vi "HEWH Round UEF.vi"(11 "Unrounded Value":dbl) -> (3 "Rounded Value":dbl format="%_3g")   [LabVIEW 2023]
panel:
  out "output variable":dbl
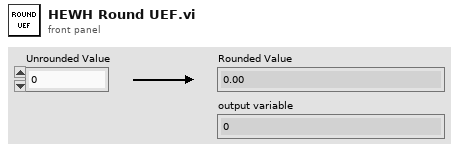
[diagram p1: front panel]
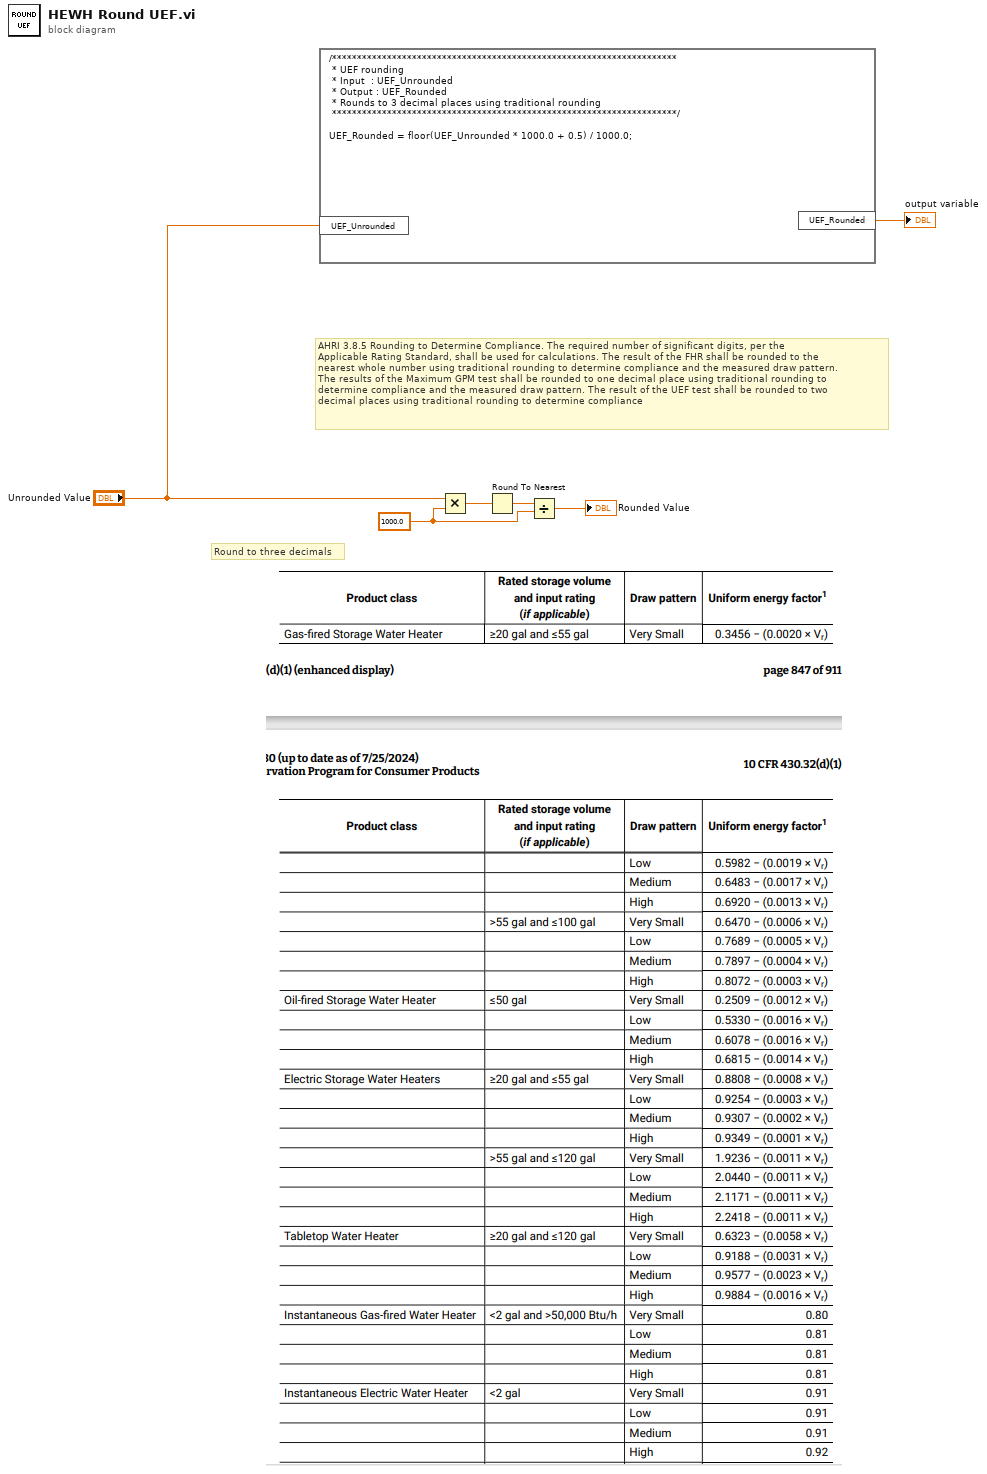
[diagram p0: block diagram]
diagram:
  w3 = 1000.0 ("y")
  # "Round to three decimals"
  # "AHRI 3.8.5 Rounding to Determine Compliance. The required number of significant digits, per the \nApplicable Rating Standard, shall be used for calculations. The result of the FHR shall be rounded to the \nnearest whole number using traditional rounding to determine compliance and the measured draw pattern. \nThe results of the Maximum GPM test shall be rounded to one decimal place using traditional rounding to \ndetermine compliance and the measured draw pattern. The result of the UEF test shall be rounded to two \ndecimal places using traditional rounding to determine compliance"
  n1 = formula code="/*********************************************************************\n * UEF rounding\n * Input  : UEF_Unrounded\n * Output : UEF_Rounded\n * Rounds to 3 decimal places using traditional rounding\n *********************************************************************/\n\nUEF_Rounded = floor(UEF_Unrounded * 1000.0 + 0.5) / 1000.0;"("UEF_Unrounded"="Unrounded Value") -> ("UEF_Rounded"=→"output variable":dbl)
  n2 = Multiply(x="Unrounded Value", y=w3) -> (x*y=w5:dbl)
  n3 = Round To Nearest(number=w5) -> (nearest integer value=w4:dbl)
  n4 = Divide(x=w4, y=w3) -> (x/y=→"Rounded Value":dbl)
